vi "Constants.vi"() -> ()   [LabVIEW 2026, in "WebPage Addon Shared.lvlib"]
doc: "Use this Global VI to access the GUIDs assigned to the page resources of the Custom Device."
uses:
  WebPage Addon Shared.lvlib
panel:
  in  "Tab Control":enum32{"GUIDs", "Constants", "Properties"}(tab)
  in  "WebPage-Custom-Device-Disable":string="5F723691-027A-41FF-9930-77045F19C5F0"
  in  "WebPage-Custom-Device":string="61c42cce-7210-4013-8cc7-f6e7840422ea"
  in  "Compiled.Settings":string="Compiled.Settings"
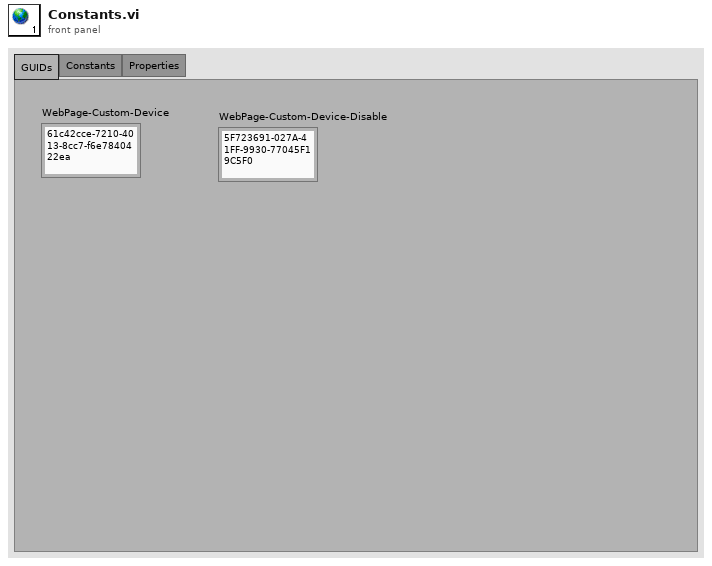
[diagram p1: front panel]
diagram:
